vi "setCRC.vi"(8 "error in (no error)":errorcluster, 11 "FixedFrameBuilder in":refnum<class "FixedFrameBuilder.lvclass">) -> (0 "error out":errorcluster, 3 "FixedFrameBuilder out":refnum<class "FixedFrameBuilder.lvclass">)   [LabVIEW 2016, in "RTModbus.lvlib" / "FixedFrameBuilder.lvclass"]
uses:
  FixedFrameBuilder.lvclass
  FixedFrameBuilder.lvclass/FixedFrameBuilder.ctl
  Common_RT_Utilities/U8ArrayBuilderManualIndexing/U8ArrayBuilderManualIndexing.lvclass
  Common_RT_Utilities/CRC16/CRC16.lvclass
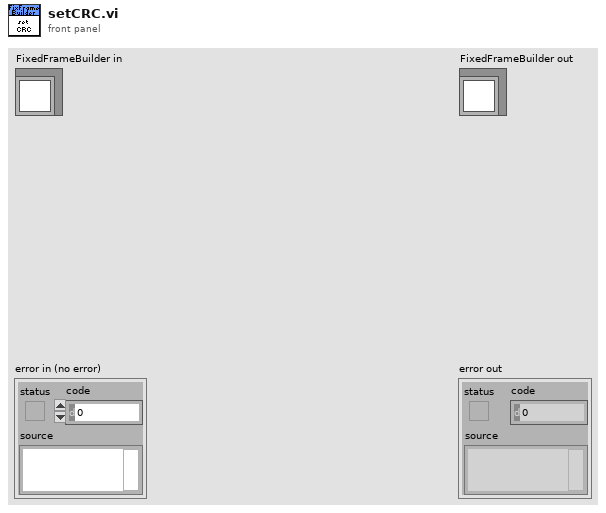
[diagram p1: front panel]
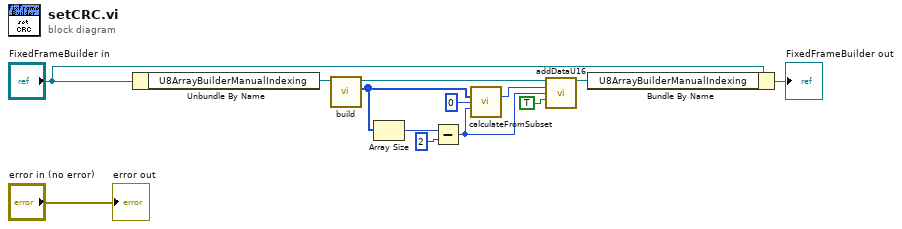
[diagram p0: block diagram]
diagram:
  n1 = Unbundle By Name("FixedFrameBuilder in") -> ("U8ArrayBuilderManualIndexing"=w7:refnum<class "U8ArrayBuilderManualIndexing.lvclass">)
  n2 = call "build.vi"("U8ArrayBuilderManualIndexing in"=w7) -> ("Array"=w6:u8[], "U8ArrayBuilderManualIndexing out"=w5:refnum<class "U8ArrayBuilderManualIndexing.lvclass">)  [unwired: 8 in, 1 out]
  n3 = Array Size(array=w6) -> (size(s)=w12:i32)
  n4 = Subtract(x=w12, y=2) -> (x-y=w4:i32)
  n5 = call "calculateFromSubset.vi"("Data"=w6, "StartIndex"=0, "Length"=w4) -> ("CRC"=w3:u16)  [unwired: 10 in, 2 out]
  n6 = call "addDataU16.vi"("U8ArrayBuilderManualIndexing in"=w5, "Data"=w3, "Index"=w4, "OverrideSwapBytes"=TRUE) -> ("U8ArrayBuilderManualIndexing out"=w1:refnum<class "U8ArrayBuilderManualIndexing.lvclass">)  [unwired: 9 in, 2 out]
  n7 = Bundle By Name(cluster="FixedFrameBuilder in", "U8ArrayBuilderManualIndexing"=w1) -> (→"FixedFrameBuilder out":refnum<class "FixedFrameBuilder.lvclass">)
  "error out" <- "error in (no error)"
